vi "Read All.vi"(6 "Per Read Size":u64=1024, 8 "Error In":errorcluster, 10 "Total Read Size":u64, 11 "Channel In":refnum<class "Channel.lvclass">) -> (0 "Error Out":errorcluster, 2 "Data":u8[](array[numeric]), 3 "Channel Out":refnum<class "Channel.lvclass">)   [LabVIEW 2018, in "Toolkit.lvlib" / "Channel.lvclass"]
uses:
  Channel.lvclass
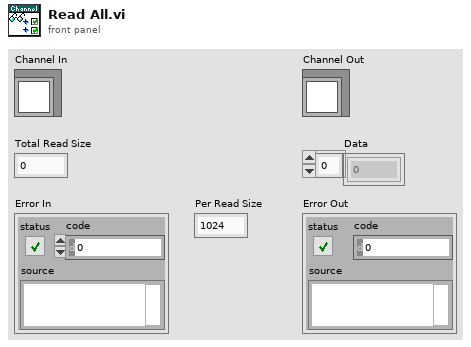
[diagram p1: front panel]
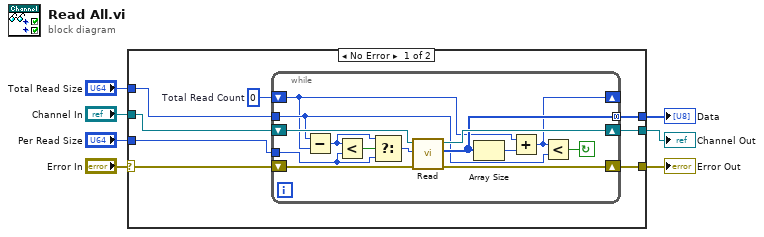
[diagram p0: block diagram]
diagram:
  n1 = case shown="No Error" "Error In" {
    selector: "Error In" -> [w8 w30]
    tunnel: "Total Read Size" -> [w14 _]
    tunnel: "Per Read Size" -> [w13 _]
    tunnel: "Channel In" -> [w12 w31]
    tunnel: [w11 _] -> w4
    tunnel: [w10 w31] -> w3
    tunnel: [w9 w30] -> w2
    frame No Error {
      w15 = u64 0  # Total Read Count
      n2 = while {
        shift-right: [w27] -> w10
        shift-left: w12 -> [w29]
        shift-right: [w26] -> w9
        shift-left: w8 -> [w28]
        tunnel: [w25] -> w11 mode=concatenating
        shift-right: [w23] -> _
        shift-left: w15 -> [w20]
        tunnel: w14 -> [w21]
        tunnel: w13 -> [w16]
        stop <- w22 continue-if-true
        n3 = Subtract(x=w21, y=w20) -> (x-y=w18:u64)
        n4 = Less?(x=w18, y=w16) -> (x < y?=w19:bool)
        n5 = Select(t=w18, s=w19, f=w16) -> (s? t:f=w17:u64)
        n6 = call "Read.vi"("Error In"=w28, "Max Data Length"=w17, "Channel In"=w29) -> ("Error Out"=w26:errorcluster, "Data"=w25:u8[], "Channel Out"=w27:refnum<class "Channel.lvclass">)  [unwired: 6 in]
        n7 = Array Size(array=w25) -> (size(s)=w24:i32)
        n8 = Add(x=w20, y=w24) -> (x+y=w23:u64)
        n9 = Less?(x=w23, y=w21) -> (x < y?=w22:bool)
      }
    }
    frame Error {
    }
  }
  "Data" <- w4
  "Channel Out" <- w3
  "Error Out" <- w2
